vi "globalSetUp.vi"(8 "error in (no error)":errorcluster, 11 "testcase-CSMSystemLevelModule.lvclass":refnum<class "testcase-CSMSystemLevelModule.lvclass">) -> (0 "error out":errorcluster, 3 "testcase-CSMSystemLevelModule.lvclass":refnum<class "testcase-CSMSystemLevelModule.lvclass">)   [LabVIEW 2017, in "testcase-CSMSystemLevelModule.lvclass"]
uses:
  testcase-CSMSystemLevelModule.lvclass
  <vilib>/addons/_JKI Toolkits/VI Tester/TestCase.llb/TestCase.lvclass
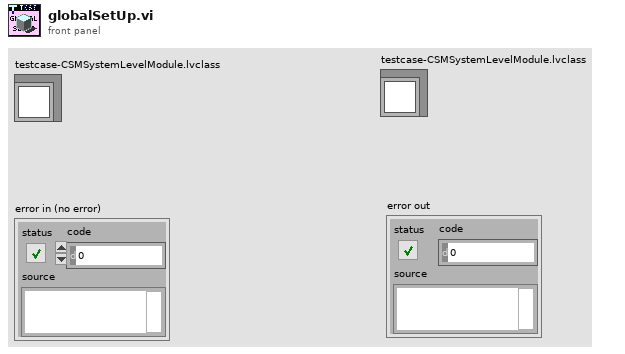
[diagram p1: front panel]
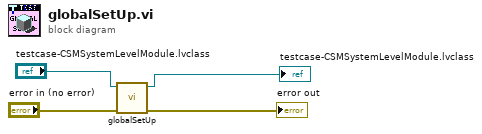
[diagram p0: block diagram]
diagram:
  n1 = call-parent "globalSetUp.vi"("error in (no error)"="error in (no error)", "TestCase in"="testcase-CSMSystemLevelModule.lvclass") -> ("error out"=→"error out":errorcluster, "TestCase out"=→"testcase-CSMSystemLevelModule.lvclass":refnum<class "testcase-CSMSystemLevelModule.lvclass">)  [unwired: 8 in]
